vi "RT Main.vi"() -> ()   [LabVIEW 2016]
panel:
  out "idle loop count":i32
  in  "Stop":bool
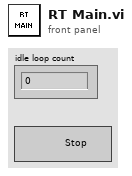
[diagram p1: front panel]
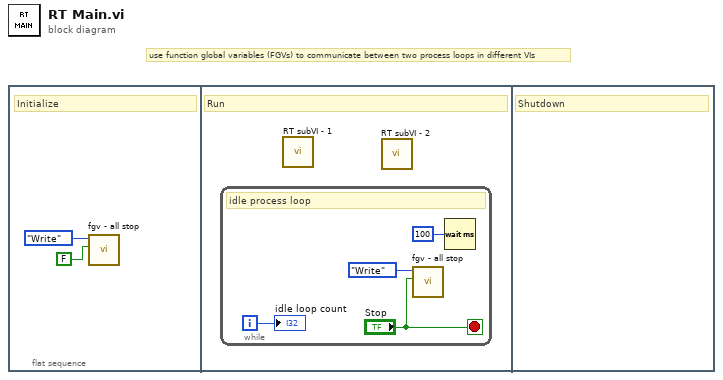
[diagram p0: block diagram]
diagram:
  # "use function global variables (FGVs) to communicate between two process loops in different VIs"
  n1 = flat-sequence {
    frame #0 {
      # "Initialize"
      n2 = call "fgv - all stop.vi"("Write Data (F)"=FALSE ("all stop"), "Operation"=enum16{"Read", "Write"}."Write") -> ()  [unwired: 8 in, 2 out]
    }
    frame #1 {
      # "Run"
      n3 = while {
        i -> [w5]
        stop <- "Stop" stop-if-true
        # "idle process loop"
        n4 = call "fgv - all stop.vi"("Write Data (F)"="Stop", "Operation"=enum16{"Read", "Write"}."Write") -> ()  [unwired: 8 in, 2 out]
        n5 = Wait (ms)(milliseconds to wait=u32 100) -> ()  [unwired: 1 out]
        "idle loop count" <- w5
      }
      n6 = call "RT subVI - 1.vi"() -> ()  [unwired: 12 in]
      n7 = call "RT subVI - 2.vi"() -> ()  [unwired: 12 in]
    }
    frame #2 {
      # "Shutdown"
    }
  }
